vi "Instr_Read 1.vi"() -> ()   [LabVIEW 2013]
doc: "Use this template to parse data you acquired from an instrument and write the data to a file.\nNote: LabVIEW enables automatic error handling by default for VIs you create from this template."
panel:
  out "record(s)":T1
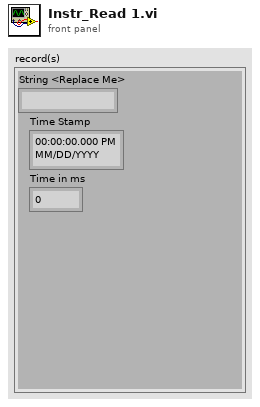
[diagram p1: front panel]
types:
  T1 = cluster{"String <Replace Me>":string, "Time Stamp":timestamp, "Time in ms":dbl}
  T2 = enum16{"open", "replace", "create", "open or create", "replace or create", "replace or create with confirmation"}
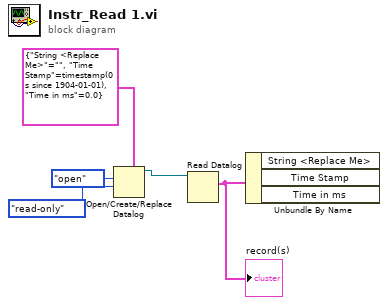
[diagram p0: block diagram]
diagram:
  n1 = Open/Create/Replace Datalog(5:T1 {"String <Replace Me>"="", "Time Stamp"=timestamp(0 s since 1904-01-01), "Time in ms"=0.0} ("Data"), 9:enum16{"read/write", "read-only", "write-only"}."read-only" ("access (0:read/write)"), 10:T2."open" ("operation (0:open)")) -> (3:w2:refnum<k1>)  [unwired: 3 in, 2 out]
  n2 = Read Datalog(7:w2) -> (2:w1:T1)  [unwired: 2 in, 2 out]
  "record(s)" <- w1
  n3 = Unbundle By Name(w1) -> ()  [unwired: 3 out]
